vi "example_LVUSBRH2_1.vi"() -> ()   [LabVIEW 2020]
uses:
  <vilib>/Instr/_visa.llb/VISA Flush IO Buffer Mask.ctl
  <vilib>/Instr/_visa.llb/VISA Configure Serial Port (Instr).vi
panel:
  out "RHumidity(%)":dbl(slide) scale=0.0..100.0
  out "Thermometer(C)":dbl(slide) scale=0.0..100.0
  in  "Btn stop":bool
  in  "VISA resource name":refnum<visa-resource-name>="COM1"
  # "Example1: Get Temperature and RHumidty data From USBRH2"
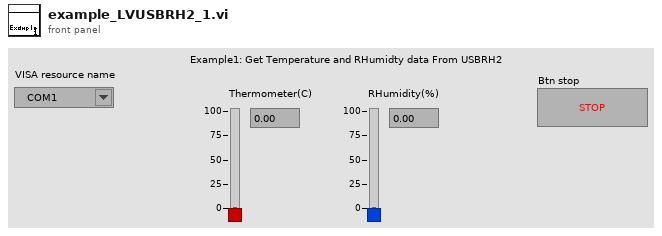
[diagram p1: front panel]
types:
  T1 = typedef "VISA Flush IO Buffer Mask.ctl" = u16
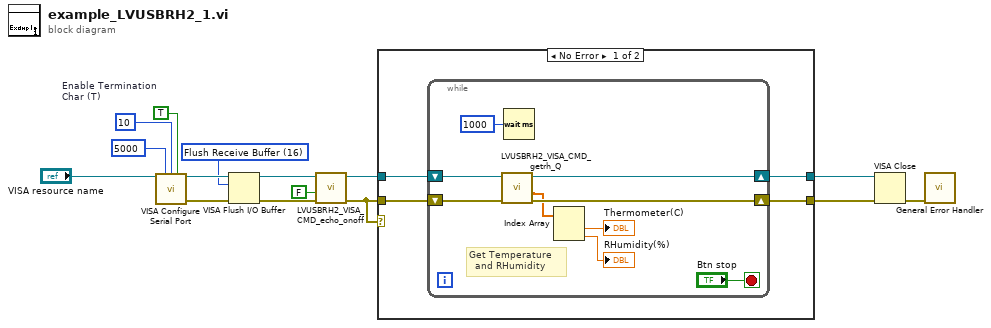
[diagram p0: block diagram]
diagram:
  w2 = T1 16 items=["Flush Receive Buffer"=16, "Write Transmit Buffer to Device"=32, "Flush Receive Buffer (No I/O)"=64, "Flush Transmit Buffer"=128] ("Mask")
  w14 = TRUE  # Enable Termination Char (T)
  n1 = call-poly "VISA Configure Serial Port"("VISA resource name"="VISA resource name", "timeout (10sec)"=u32 5000, "termination char\n(0xA = '\\n' = LF)"=u8 10 ("termination char\n(0xA = '\\n' = LF)"), "Enable Termination\nChar (T)"=w14) -> ("VISA resource name out"=w7:refnum<visa-resource-name>, "error out"=w8:errorcluster)  [unwired: 10 in]
  n2 = VISA Flush I/O Buffer(VISA resource name=w7, mask (16)=w2) -> (VISA resource name out=w3:refnum<visa-resource-name>)  [unwired: 1 in, 1 out]
  n3 = call "LVUSBRH2_VISA_CMD_echo_onoff.vi"("error in (no error)"=w8, "echo on/off)(F)"=FALSE, "VISA rssc"=w3) -> ("error out"=w5:errorcluster, "VISA rssc out"=w6:refnum<visa-resource-name>)  [unwired: 7 in]
  n4 = case shown="No Error" w5 {
    tunnel: w6 -> [w18 w29]
    tunnel: w5 -> [w17 w28]
    tunnel: [w16 w29] -> w12
    tunnel: [w15 w28] -> w11
    frame No Error {
      n5 = while {
        shift-right: [w25] -> w16
        shift-left: w18 -> [w27]
        shift-right: [w24] -> w15
        shift-left: w17 -> [w26]
        stop <- "Btn stop" stop-if-true
        # "Get Temperature\n  and RHumidity"
        n6 = call "LVUSBRH2_VISA_CMD_getrh_Q.vi"("error in (no error)"=w26, "VISA rssc"=w27) -> ("error out"=w24:errorcluster, "data[]"=w21:dbl[], "VISA rssc out"=w25:refnum<visa-resource-name>)  [unwired: 7 in]
        n7 = Wait (ms)(milliseconds to wait=u32 1000) -> ()  [unwired: 1 out]
        n8 = Index Array(array=w21) -> (element #1=→"Thermometer(C)":dbl, element #2=→"RHumidity(%)":dbl)  [unwired: 2 in]
      }
    }
    frame Error {
    }
  }
  n9 = VISA Close(VISA resource name=w12, error in (no error)=w11) -> (error out=w9:errorcluster)
  n10 = call <vilib>:"General Error Handler.vi"("error in (no error)"=w9) -> ()  [unwired: 10 in, 5 out]
